vi "open aux joystick.vi"   [LabVIEW 2019]
uses:
  <vilib>/Rock Robotics/WPI/Utilities/WPI_GetSetVariantRefNum.vi
  Robot Global Data.vi
types:
  T1 = typedef "WPI_JoystickDevRef.ctl" = cluster{"Device":T2}
  T2 = typedef "WPI_JoystickDeviceEnum.ctl" = enum16{"USB 0", "USB 1", "USB 2", "USB 3", "USB 4", "USB 5"}
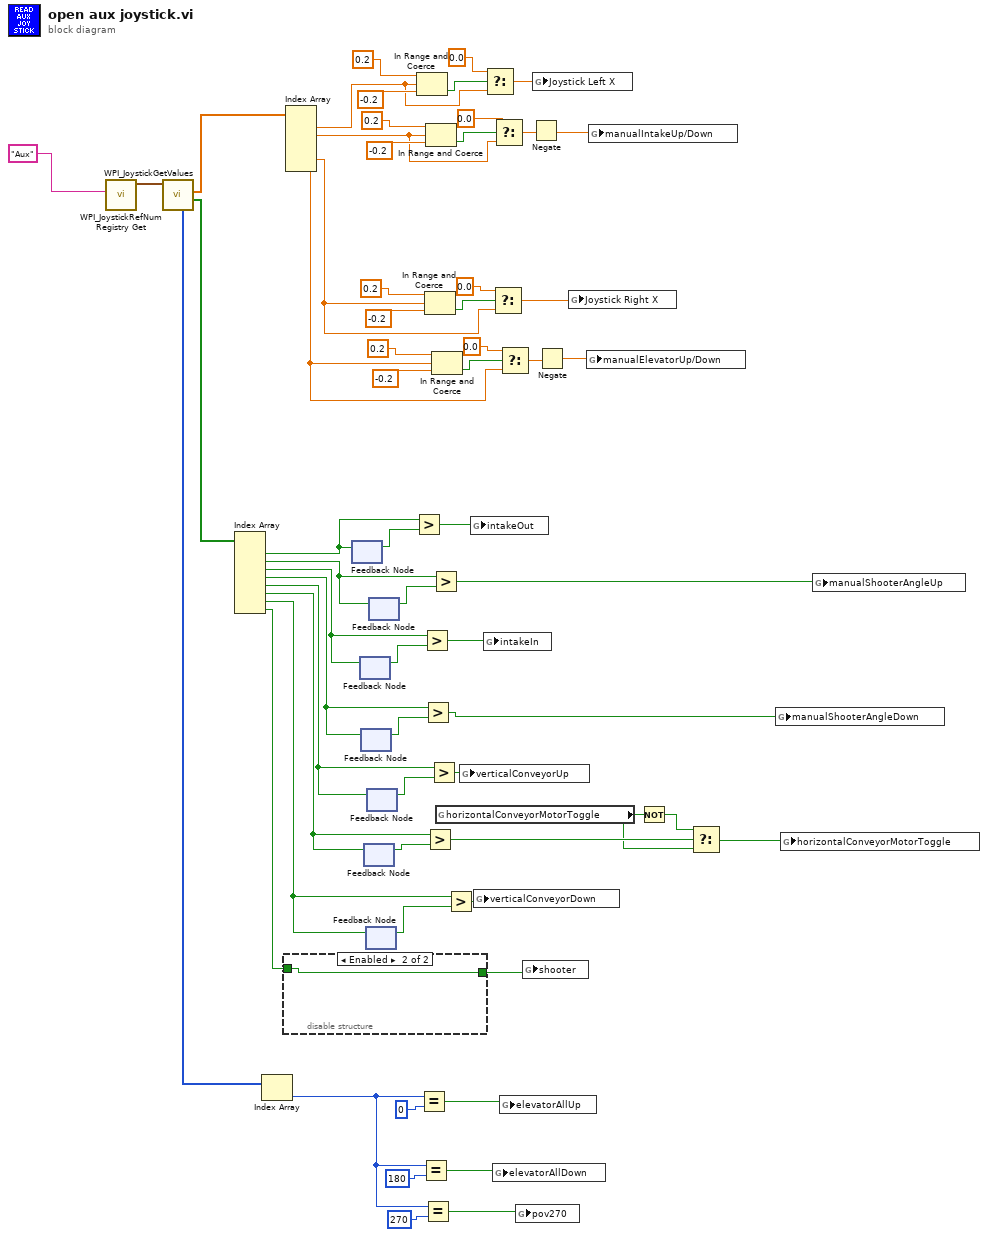
[diagram p0: block diagram]
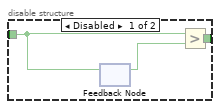
[diagram p2: hidden frame]
diagram:
  n1 = call <vilib>:"WPI_JoystickRefNum Registry Get.vi"("refnum name"="Aux") -> ("JoystickDevRef"=w63:T1)  [unwired: 9 in, 1 out]
  n2 = call <vilib>:"WPI_JoystickGetValues.vi"("JoystickDevRef"=w63) -> ("Buttons"=w61:bool[], "Axes"=w62:dbl[], "POVs"=w10:i16[])  [unwired: 6 in, 2 out]
  n3 = Index Array(array=w61) -> (element #1=w59:bool, element #2=w56:bool, element #3=w53:bool, element #4=w51:bool, element #5=w26:bool, element #6=w15:bool, element #7=w22:bool, element #8=w18:bool)  [unwired: 8 in]
  n4 = Index Array(array=w10) -> (element=w5:i16)  [unwired: 1 in]
  n5 = disable-structure shown="Enabled" {
    disable-tunnel: [w66 w68] -> w19
    disable-tunnel: w18 -> [w65 w68]
    frame Disabled {
      n6 = feedback #1() -> (w67:bool)  [unwired: 1 in]
      n7 = feedback-in #1(w65) -> ()
      n8 = Greater?(x=w65, y=w67) -> (0:w66:bool)
    }
    frame Enabled {
    }
  }
  n9 = Index Array(array=w62) -> (element #1=w45:dbl, element #2=w40:dbl, element #5=w23:dbl, element #6=w31:dbl)  [unwired: 6 in, 2 out]
  n10 = feedback #2() -> (w58:bool)  [unwired: 1 in]
  n11 = feedback-in #2(w59) -> ()
  n12 = feedback #3() -> (w54:bool)  [unwired: 1 in]
  n13 = feedback-in #3(w53) -> ()
  n14 = feedback #4() -> (w52:bool)  [unwired: 1 in]
  n15 = feedback-in #4(w51) -> ()
  n16 = feedback #5() -> (w16:bool)  [unwired: 1 in]
  n17 = feedback-in #5(w15) -> ()
  n18 = feedback #6() -> (w21:bool)  [unwired: 1 in]
  n19 = feedback-in #6(w22) -> ()
  n20 = feedback #7() -> (w27:bool)  [unwired: 1 in]
  n21 = feedback-in #7(w26) -> ()
  n22 = feedback #8() -> (w57:bool)  [unwired: 1 in]
  n23 = feedback-in #8(w56) -> ()
  n24 = Greater?(x=w59, y=w58) -> (0:w60:bool)
  n25 = In Range and Coerce(upper limit=0.2, x=w45, lower limit=-0.2) -> (In Range?=w46:bool)  [unwired: 1 out]
  n26 = Equal?(x=w5, y=i16 0) -> (x = y?=w8:bool)
  n27 = Equal?(x=w5, y=i16 180) -> (x = y?=w6:bool)
  n28 = Greater?(x=w53, y=w54) -> (0:w55:bool)
  n29 = Greater?(x=w51, y=w52) -> (0:w1:bool)
  n30 = Equal?(x=w5, y=i16 270) -> (x = y?=w3:bool)
  n31 = In Range and Coerce(upper limit=0.2, x=w23, lower limit=-0.2) -> (In Range?=w37:bool)  [unwired: 1 out]
  n32 = Greater?(x=w15, y=w16) -> (0:w14:bool)
  n33 = In Range and Coerce(upper limit=0.2, x=w40, lower limit=-0.2) -> (In Range?=w41:bool)  [unwired: 1 out]
  n34 = Greater?(x=w26, y=w27) -> (0:w28:bool)
  n35 = Greater?(x=w56, y=w57) -> (0:w2:bool)
  n36 = In Range and Coerce(upper limit=0.2, x=w31, lower limit=-0.2) -> (In Range?=w34:bool)  [unwired: 1 out]
  n37 = global read "Robot Global Data.vi" "horizontalConveyorMotorToggle"() -> (w13:bool)
  n38 = Greater?(x=w22, y=w21) -> (0:w20:bool)
  n39 = global write "Robot Global Data.vi" "verticalConveyorUp"(w28) -> ()
  n40 = global write "Robot Global Data.vi" "intakeOut"(w60) -> ()
  n41 = global write "Robot Global Data.vi" "verticalConveyorDown"(w20) -> ()
  n42 = global write "Robot Global Data.vi" "intakeIn"(w55) -> ()
  n43 = Select(t=0.0, s=w46, f=w45) -> (s? t:f=w48:dbl)
  n44 = Select(t=0.0, s=w37, f=w23) -> (s? t:f=w36:dbl)
  n45 = global write "Robot Global Data.vi" "elevatorAllDown"(w6) -> ()
  n46 = Select(t=0.0, s=w41, f=w40) -> (s? t:f=w39:dbl)
  n47 = Select(t=0.0, s=w34, f=w31) -> (s? t:f=w33:dbl)
  n48 = global write "Robot Global Data.vi" "elevatorAllUp"(w8) -> ()
  n49 = global write "Robot Global Data.vi" "pov270"(w3) -> ()
  n50 = global write "Robot Global Data.vi" "shooter"(w19) -> ()
  n51 = Negate(x=w39) -> (-x=w17:dbl)
  n52 = global write "Robot Global Data.vi" "Joystick Left X"(w48) -> ()
  n53 = Negate(x=w33) -> (-x=w32:dbl)
  n54 = global write "Robot Global Data.vi" "Joystick Right X"(w36) -> ()
  n55 = global write "Robot Global Data.vi" "manualElevatorUp/Down"(w32) -> ()
  n56 = global write "Robot Global Data.vi" "manualIntakeUp/Down"(w17) -> ()
  n57 = Not(x=w13) -> (.not. x?=w12:bool)
  n58 = Select(t=w12, s=w14, f=w13) -> (s? t:f=w11:bool)
  n59 = global write "Robot Global Data.vi" "manualShooterAngleDown"(w1) -> ()
  n60 = global write "Robot Global Data.vi" "horizontalConveyorMotorToggle"(w11) -> ()
  n61 = global write "Robot Global Data.vi" "manualShooterAngleUp"(w2) -> ()
